vi "FPGA_ThreePointSuspension.vi"() -> ()   [LabVIEW 2024]
uses:
  <vilib>/rvi/Emulation/niFpgaGetClockAttributes.vi
  <vilib>/rvi/Emulation/niFpgaSctlEmulationGetInTimedLoop.vi
  <vilib>/rvi/Emulation/niFpgaEmulationReportErrorSimple.vi
  <vilib>/rvi/Emulation/niFpgaEmulationIsFPGAContextNoSignature.vi
  <vilib>/rvi/DataTransferAndStorage/Container/Common/niFpgaContainerGetUniqueNameForEmu.vi
  <vilib>/rvi/Memory/Memory_Emulation/niFpgaMemoryEmulationCacheClearOnFirstRun.vi
  <vilib>/rvi/Memory/Memory_Emulation/nirvimemoryEmulationManagerCache_MakeExclusive.vi
  <vilib>/rvi/Memory/Memory_Emulation/niFpgaMemoryEmulationValidateCache.vi
  <vilib>/rvi/Memory/Memory_Emulation/nirvimemoryEmulationManagerCache_InsertValue.vi
  <vilib>/Utility/error.llb/Clear Errors.vi
  <vilib>/rvi/Memory/Memory_Emulation/nirvimemoryEmulationManagerCache_ReleaseExclusive.vi
  <vilib>/rvi/Memory/Memory_Emulation/nirvimemoryEmulationManagerCache_GetValue.vi
  <vilib>/rvi/Memory/Memory_Emulation/nirvimemoryEmulationManagerCache_SetValue.vi
  <vilib>/rvi/Emulation/niFpgaProcessEmulError.vi
  <vilib>/rvi/Emulation/niFpgaCriticalErrorInLSC.vi
  <vilib>/rvi/eio/common/nirviEmuTemplateMethod_errors.vi
  <vilib>/eio/utilities/niEioResolveVilibRelativePath.vi
  <vilib>/rvi/interface/RandomDataEmulation/niFpgaRandomDataHandleErrors.vi
  <vilib>/rvi/DataTransferAndStorage/Container/XNode/niFpgaContainer.xnode
  <vilib>/rvi/DataTransferAndStorage/Register/Emulation/niFpgaRegisterEmulation.vi
  <vilib>/eio/EIONode/EIONode.xnode
  <vilib>/rvi/interface/RandomDataEmulation/nirviRandomDataFpgaReadWriteTemplate.vi
  <vilib>/rvi/FXPMathLib/FxpSub/XNode/nifxpmath_Sub.xnode
  <vilib>/rvi/FXPMathLib/sim/FxpSim.dll
panel:
  in  "X_End":fxp<+/-,48,16>
  in  "Y_End":fxp<+/-,48,16>
  in  "stop":bool
  in  "RetRate us":i32
  in  "AppRate us":i32
  in  "Retract":fxp<+/-,48,16>
  in  "Y_Start":fxp<+/-,48,16>
  in  "X_Start":fxp<+/-,48,16>
  in  "Threshold":fxp<+/-,48,16>
  out "TargetDone?":bool
  out "ScanFinished?":bool
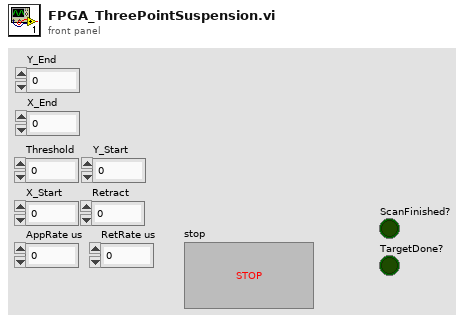
[diagram p1: front panel]
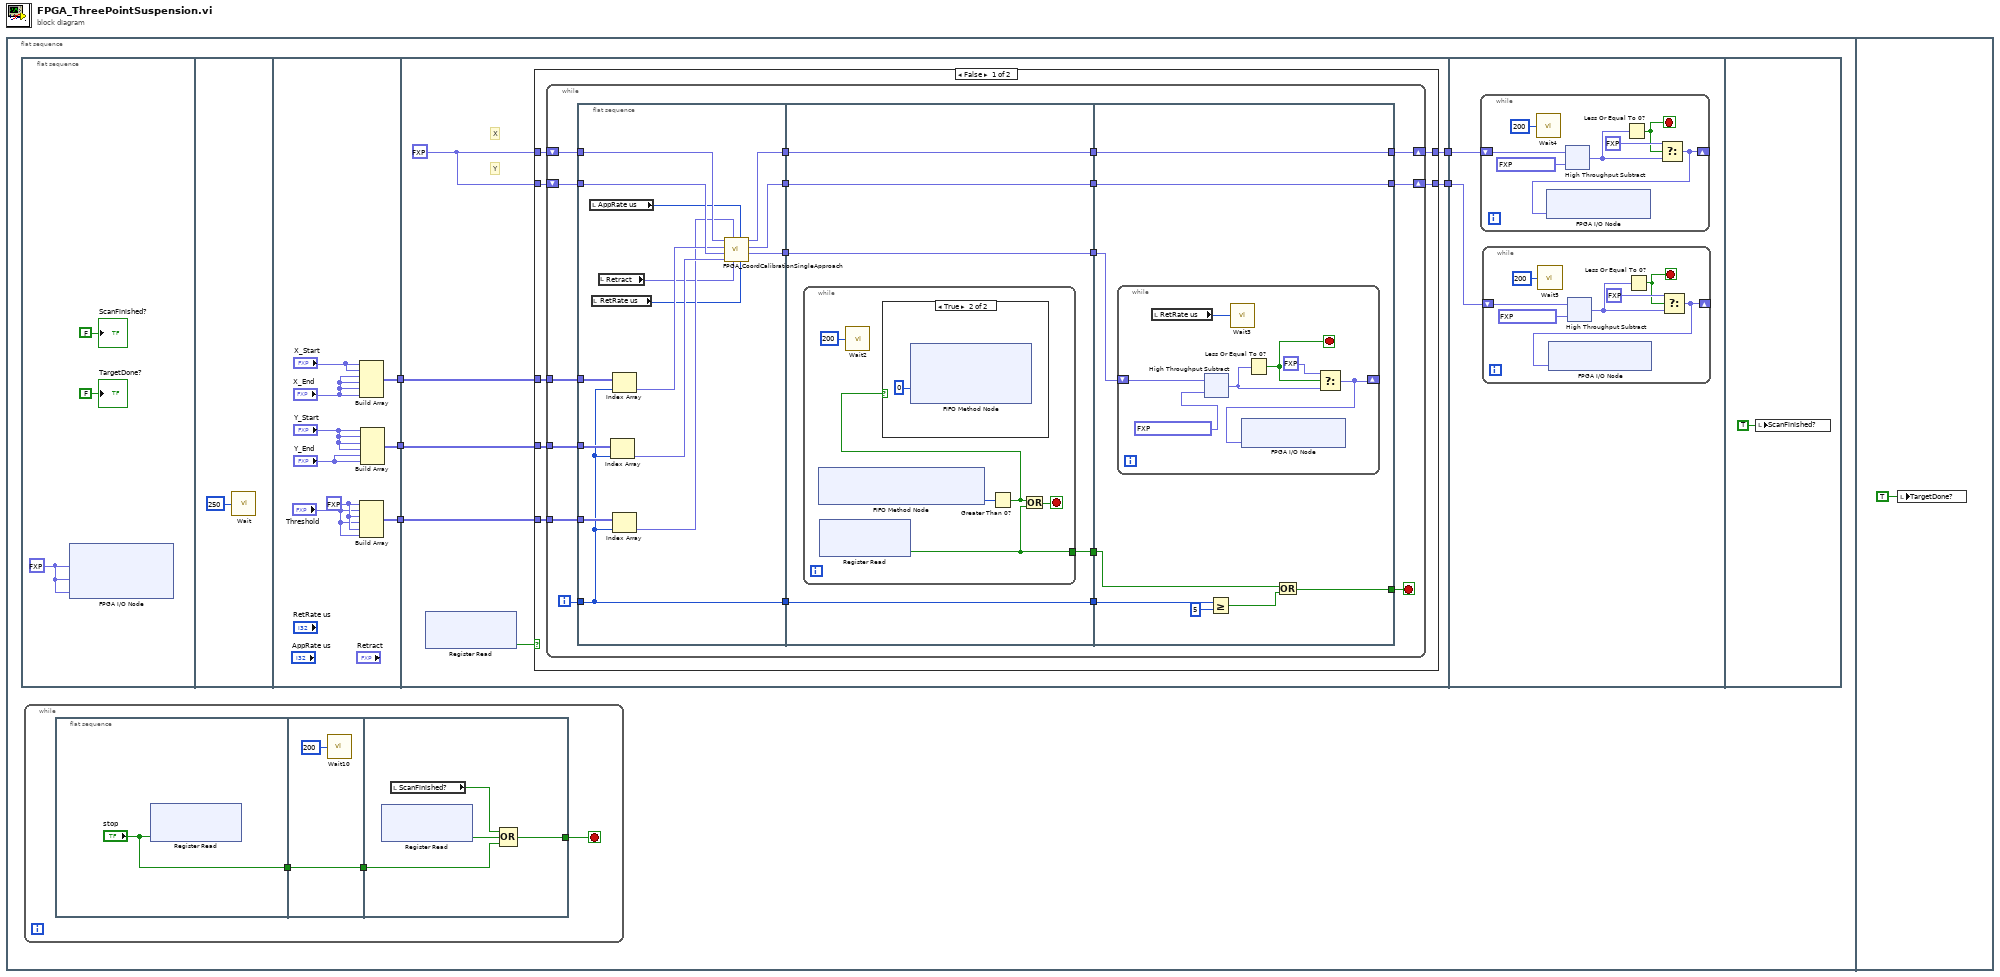
[diagram p0: block diagram]
diagram:
  n1 = flat-sequence {
    frame #0 {
      n2 = flat-sequence {
        tunnel: [w22] -> w5
        tunnel: [w21] -> w4
        tunnel: [w20] -> w3
        tunnel: w5 -> [w34]
        tunnel: w4 -> [w33]
        tunnel: w3 -> [w32]
        tunnel: [w30] -> w2
        tunnel: [w29] -> w1
        tunnel: w2 -> [w105]
        tunnel: w1 -> [w104]
        frame #0 {
          w18 = fxp<+/-,20,5> 0.0 ("Connector0/AO0")
          n3 = xnode "FPGA I/O Node"("Connector0/AO0"=w18, "Connector0/AO1"=w18, "Connector0/AO2"=w18) -> ()  [unwired: 3 in, 3 out]
          "ScanFinished?" <- FALSE
          "TargetDone?" <- FALSE
        }
        frame #1 {
          n4 = call "Wait"("Count(mSec)"=u8 250) -> ()  [unwired: 1 out]
        }
        frame #2 {
          w24 = fxp<+/-,48,16> 0.0 ("element")
          n5 = Build Array("X_Start", "X_Start", "X_End", "X_End", "X_End", "X_End") -> (w22:fxp<+/-,48,16>[])
          n6 = Build Array(w24, "Threshold", w24, "Threshold", w24, "Threshold") -> (w20:fxp<+/-,48,16>[])
          n7 = Build Array("Y_Start", "Y_Start", "Y_Start", "Y_Start", "Y_End", "Y_End") -> (w21:fxp<+/-,48,16>[])
        }
        frame #3 {
          w31 = fxp<+/-,48,16> 0.0 ("element")
          # "Y"
          # "X"
          n8 = xnode ("Register Read")() -> ("Data"=w35:bool)  [unwired: 1 in, 1 out]
          n9 = case shown="False" w35 {
            tunnel: w34 -> [w42 _]
            tunnel: w33 -> [w41 _]
            tunnel: w32 -> [w40 _]
            tunnel: w31 -> [w39 w103]
            tunnel: w31 -> [w38 w102]
            tunnel: [w37 w103] -> w30
            tunnel: [w36 w102] -> w29
            frame False {
              n10 = while {
                tunnel: w42 -> [w56]
                tunnel: w41 -> [w55]
                tunnel: w40 -> [w54]
                shift-right: [w49] -> w37
                shift-left: w39 -> [w53]
                shift-right: [w46] -> w36
                shift-left: w38 -> [w52]
                i -> [w59]
                stop <- w57 stop-if-true
                n11 = flat-sequence {
                  tunnel: [w70] -> w60
                  tunnel: w59 -> [w70]
                  tunnel: w56 -> [w73]
                  tunnel: w55 -> [w72]
                  tunnel: w54 -> [w71]
                  tunnel: w53 -> [w75]
                  tunnel: w52 -> [w74]
                  tunnel: [w63] -> w51
                  tunnel: [w62] -> w48
                  tunnel: [w61] -> w45
                  tunnel: w60 -> [w80]
                  tunnel: [w80] -> w58
                  tunnel: w51 -> [w79]
                  tunnel: [w79] -> w50
                  tunnel: w48 -> [w78]
                  tunnel: [w78] -> w47
                  tunnel: w45 -> [w77]
                  tunnel: [w77] -> w44
                  tunnel: [w76] -> w43
                  tunnel: w58 -> [w94]
                  tunnel: [w88] -> w57
                  tunnel: w50 -> [w92]
                  tunnel: [w92] -> w49
                  tunnel: w47 -> [w91]
                  tunnel: [w91] -> w46
                  tunnel: w44 -> [w87]
                  tunnel: w43 -> [w90]
                  frame #0 {
                    n12 = local read "AppRate us"() -> (w66:i32)
                    n13 = local read "RetRate us"() -> (w64:i32)
                    n14 = local read "Retract"() -> (w65:fxp<+/-,48,16>)
                    n15 = Index Array(array=w72, index=w70) -> (element=w68:fxp<+/-,48,16>)
                    n16 = Index Array(array=w73, index=w70) -> (element=w69:fxp<+/-,48,16>)
                    n17 = Index Array(array=w71, index=w70) -> (element=w67:fxp<+/-,48,16>)
                    n18 = call "FPGA_CoordCalibrationSingleApproach.vi"("RetRate us"=w64, "AppRate us"=w66, "Retract"=w65, "Threshold"=w67, "Y_Dst"=w68, "Y_Start"=w74, "X_Dst"=w69, "X_Start"=w75) -> ("Z_Out"=w61:fxp<+/-,48,16>, "Y_Out"=w62:fxp<+/-,48,16>, "X_Out"=w63:fxp<+/-,48,16>)  [unwired: 1 in]
                  }
                  frame #1 {
                    n19 = while {
                      tunnel: [w81] -> w76
                      stop <- w82 stop-if-true
                      n20 = xnode ("FIFO Method Node")() -> ("Number of Elements to Read"=w85:u32)  [unwired: 1 in, 1 out]
                      n21 = xnode ("Register Read")() -> ("Data"=w81:bool)  [unwired: 1 in, 1 out]
                      n22 = call "Wait2"("Count(uSec)"=u8 200) -> ()  [unwired: 1 out]
                      n23 = Greater Than 0?(x=w85) -> (x > 0?=w84:bool)
                      n24 = case shown="True" w84 {
                        frame False {
                        }
                        frame True {
                          n25 = xnode ("FIFO Method Node")("Timeout"=0) -> ()  [unwired: 1 in, 3 out]
                        }
                      }
                      n26 = Or(x=w84, y=w81) -> (x .or. y?=w82:bool)
                    }
                  }
                  frame #2 {
                    n27 = while {
                      shift-right: [w97] -> _
                      shift-left: w87 -> [w100]
                      stop <- w96 stop-if-true
                      n28 = local read "RetRate us"() -> (w101:i32)
                      n29 = xnode "High Throughput Subtract"("x"=w100, "y"=fxp<+/-,48,16> 0.00030517578125) -> ("x-y"=w98:fxp<+/-,48,16>)
                      n30 = call "Wait3"("Count(uSec)"=w101) -> ()  [unwired: 1 out]
                      n31 = Less Or Equal To 0?(x=w98) -> (x <= 0?=w96:bool)
                      n32 = Select(t=fxp<+/-,48,16> 0.0, s=w96, f=w98) -> (s? t:f=w97:fxp<+/-,48,16>)
                      n33 = xnode "FPGA I/O Node"("Connector0/AO2"=w97) -> ()  [unwired: 1 in, 1 out]
                    }
                    n34 = Greater Or Equal?(x=w94, y=5) -> (x >= y?=w89:bool)
                    n35 = Or(x=w90, y=w89) -> (x .or. y?=w88:bool)
                  }
                }
              }
            }
            frame True {
            }
          }
        }
        frame #4 {
          n36 = while {
            shift-right: [w113] -> _
            shift-left: w105 -> [w119]
            stop <- w116 stop-if-true
            n37 = call "Wait4"("Count(uSec)"=u32 200) -> ()  [unwired: 1 out]
            n38 = xnode "High Throughput Subtract"("x"=w119, "y"=fxp<+/-,48,16> 0.0048828125) -> ("x-y"=w115:fxp<+/-,48,16>)
            n39 = Less Or Equal To 0?(x=w115) -> (x <= 0?=w116:bool)
            n40 = Select(t=fxp<+/-,48,16> 0.0, s=w116, f=w115) -> (s? t:f=w113:fxp<+/-,48,16>)
            n41 = xnode "FPGA I/O Node"("Connector0/AO0"=w113) -> ()  [unwired: 1 in, 1 out]
          }
          n42 = while {
            shift-right: [w106] -> _
            shift-left: w104 -> [w112]
            stop <- w109 stop-if-true
            n43 = call "Wait5"("Count(uSec)"=u32 200) -> ()  [unwired: 1 out]
            n44 = xnode "High Throughput Subtract"("x"=w112, "y"=fxp<+/-,48,16> 0.0048828125) -> ("x-y"=w108:fxp<+/-,48,16>)
            n45 = Less Or Equal To 0?(x=w108) -> (x <= 0?=w109:bool)
            n46 = Select(t=fxp<+/-,48,16> 0.0, s=w109, f=w108) -> (s? t:f=w106:fxp<+/-,48,16>)
            n47 = xnode "FPGA I/O Node"("Connector0/AO1"=w106) -> ()  [unwired: 1 in, 1 out]
          }
        }
        frame #5 {
          n48 = local write "ScanFinished?"(TRUE ("ScanFinished?")) -> ()
        }
      }
      n49 = while {
        stop <- w6 stop-if-true
        n50 = flat-sequence {
          tunnel: ["stop"] -> w7
          tunnel: [w10] -> w8
          tunnel: w7 -> [w10]
          tunnel: w8 -> [w13]
          tunnel: [w12] -> w6
          frame #0 {
            n51 = xnode ("Register Read")("Data"="stop") -> ()  [unwired: 1 in, 1 out]
          }
          frame #1 {
            n52 = call "Wait10"("Count(uSec)"=u8 200) -> ()  [unwired: 1 out]
          }
          frame #2 {
            n53 = xnode ("Register Read")() -> ("Data"=w15:bool)  [unwired: 1 in, 1 out]
            n54 = local read "ScanFinished?"() -> (w14:bool)
            n55 = Compound Arithmetic op=OR(w14, w15, w13) -> (w12:bool)
          }
        }
      }
    }
    frame #1 {
      n56 = local write "TargetDone?"(TRUE ("ScanFinished?")) -> ()
    }
  }
